vi "FXP NIPLL_VCO.vi"(9 "nominal freq [U16.0]":fxp<+,16,0>, 10 "Kv [U16.0]":fxp<+,16,0>, 11 "v [I48.17]":fxp<+/-,48,17>) -> (0 "f":fxp<+/-,32,0> format="%.32g", 1 "z [I32.1]":fxp<+/-,32,1>, 2 "sin(z) [I16.2]":fxp<+/-,16,2> format="%.15g", 3 "cos(z) [I16.2]":fxp<+/-,16,2> format="%.15g")   [LabVIEW 2012]
uses:
  <vilib>/Platform/TimedLoop/XDataNode/timing_clust.ctl
  <vilib>/Platform/TimedLoop/XDataNode/nitl_modes.ctl
  <vilib>/Platform/TimedLoop/XDataNode/wakeup.ctl
  <vilib>/rvi/FXPMathLib/FxpConvert/subVIs/nifxpmath_Convert_SimConfig.ctl
  <vilib>/fxp/LVFixedPointQuantizationPolicyTypeDef.ctl
  <vilib>/fxp/LVFixedPointOverflowPolicyTypeDef.ctl
  <vilib>/rvi/FXPMathLib/basic elements/FxpIntAccumulator/subVIs/nifxpmath_IntAccumulator_SimConfig.ctl
  <vilib>/rvi/FXPMathLib/FxpSinAndCos/subVIs/nifxpmath_SinAndCos_SimConfig.ctl
  <vilib>/rvi/Emulation/niFpgaSctlEmulationRegisterWithScheduler.vi
  <vilib>/rvi/FXPMathLib/FxpConvert/simVIs/DllFxpConvertTemp_sub.vi
  <vilib>/rvi/FXPMathLib/basic elements/FxpIntAccumulator/simVIs/DllFxpIntAccumulator_sub.vi
  <vilib>/rvi/Emulation/niFpgaSctlEmulationScheduler.vi
  <vilib>/rvi/FXPMathLib/FxpSinAndCos/simVIs/DllFxpSinAndCosTemp_sub.vi
  <vilib>/Platform/TimedLoop/XDataNode/XDataNode.xnode
  <vilib>/rvi/FXPMathLib/FxpConvert/XNode/nifxpmath_Convert.xnode
  <vilib>/rvi/FXPMathLib/FxpMul/XNode/nifxpmath_Multiplier.xnode
  <vilib>/rvi/FXPMathLib/FxpAdd/XNode/nifxpmath_Add.xnode
  <vilib>/rvi/FXPMathLib/basic elements/FxpIntAccumulator/XNode/nifxpmath_IntAccumulator.xnode
  <vilib>/rvi/FXPMathLib/FxpSinAndCos/XNode/nifxpmath_SinAndCos.xnode
  <vilib>/rvi/FXPMathLib/sim/FxpSim.dll
  <vilib>/Platform/TimedLoop/XDataNode/XDNodeRunTimeDep.lvlib
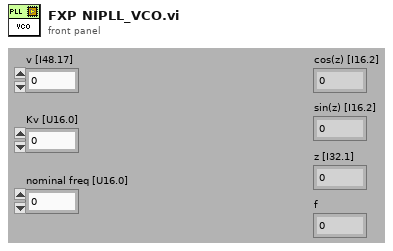
[diagram p1: front panel]
types:
  T1 = typedef "XDNodeRunTimeDep.lvlib/timing_clust.ctl" = cluster{"Expected End [f-1]":u64, "Actual End [f-1]":u64, "Finished Late? [f-1]":bool, "Expected End [i-1]":u64, "Actual End [i-1]":u64, "Finished Late? [i-1]":bool, "Expected Start [i]":u64, "Actual Start [i]":u64, "Expected Start [f]":u64, "Actual Start [f]":u64, "Source Name":string, "Structure Name":string, "Period":i64, "Deadline":i64, "Offset":i64, "Start":i64, "Priority":i32, "Timeout":i32, "Mode":T2, "Wakeup Reason":T3, "Error":errorcluster, "Source Type":string, "Secondary Source Type":string, "Global End Time":u64, "Global Start Time":u64, "Frame Duration":u64, "Iteration Duration":u64, "Assigned CPU":i32, "I/O Scan Engine Mode":u32}
  T2 = typedef "XDNodeRunTimeDep.lvlib/nitl_modes.ctl" = enum32{"No Change", "Process missed periods, maintain original phase", "Discard missed periods, maintain original phase", "Process missed periods, ignore original phase", "Discard missed periods, ignore original phase"}
  T3 = typedef "XDNodeRunTimeDep.lvlib/wakeup.ctl" = enum32{"Normal", "Aborted", "Asynchronous wakeup", "Timing source error", "Timed loop error", "Timeout"}
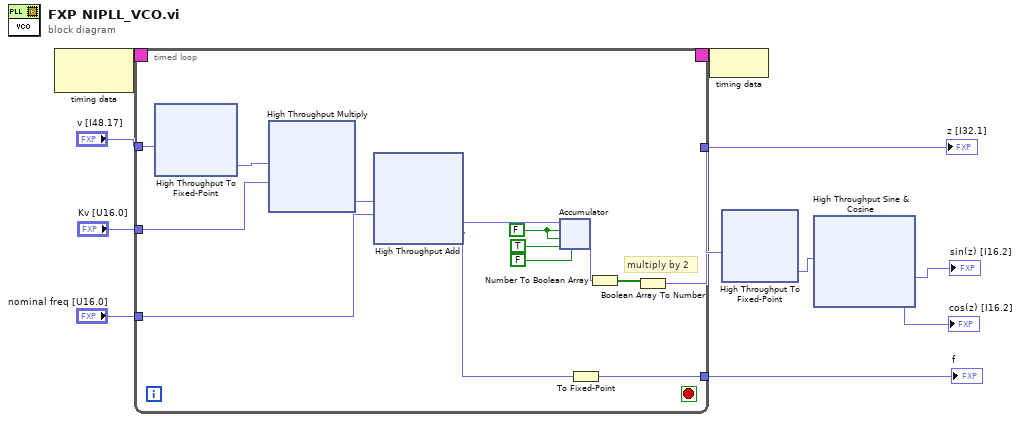
[diagram p0: block diagram]
diagram:
  n1 = node-c288() -> (w2:T1)  [unwired: 1 in]
  n2 = timed-loop {
    timing: w2 -> [_]
    timing-out: [_] -> w1
    tunnel: "Kv [U16.0]" -> [w23]
    tunnel: "nominal freq [U16.0]" -> [w22]
    tunnel: [w21] -> w6
    tunnel: "v [I48.17]" -> [w14]
    tunnel: [w11] -> w4
    stop <- _ stop-if-true
    w20 = FALSE ("is sub")
    # "multiply by 2"
    n3 = xnode ("High Throughput To Fixed-Point")("x"=w14) -> ("y"=w13:fxp<+/-,32,17>)
    n4 = xnode ("High Throughput Multiply")("x"=w13, "y"=w23) -> ("x*y"=w17:fxp<+/-,32,0>)
    n5 = xnode ("High Throughput Add")("x"=w17, "y"=w22) -> ("x+y"=w15:fxp<+/-,32,0>)
    n6 = xnode "Accumulator"("x"=w15, "load (F)"=w20, "is sub? (F)"=w20, "enable (T)"=TRUE ("enable"), "carry-in/inverted borrow-in (F)"=FALSE ("cin/nbin")) -> ("s"=w12:fxp<+/-,32,0>)  [unwired: 1 out]
    n7 = To Fixed-Point(number=w15) -> (fixed-point=w21:fxp<+/-,32,0>)  [unwired: 1 in]
    n8 = Number To Boolean Array(number=w12) -> (Boolean array=w16:bool[])
    n9 = Boolean Array To Number(Boolean array=w16) -> (number=w11:fxp<+/-,32,1>)
  }
  "z [I32.1]" <- w4
  "f" <- w6
  n10 = node-c288(w1) -> ()
  n11 = xnode ("High Throughput To Fixed-Point")("x"=w4) -> ("y"=w3:fxp<+/-,16,1>)
  n12 = xnode "High Throughput Sine & Cosine"("x (pi)"=w3) -> ("sin(x)"=→"sin(z) [I16.2]":fxp<+/-,16,2>, "cos(x)"=→"cos(z) [I16.2]":fxp<+/-,16,2>)
